vi "TestResult.vi"(0 "Name":string, 1 "Value":string, 2 "StandardValue":string, 3 "Unit":string, 4 "LowerLimit":string, 5 "UpperLimit":string, 6 "Status":T2(ring), 7 "Result":string, 8 "ProductName":string, 10 "toolID":string) -> (14 "TestIteams":T1[](array[typedef]), 15 "TestIteams2":T1[](array[typedef]))   [LabVIEW 2024]
uses:
  Ctr/TestItems.ctl
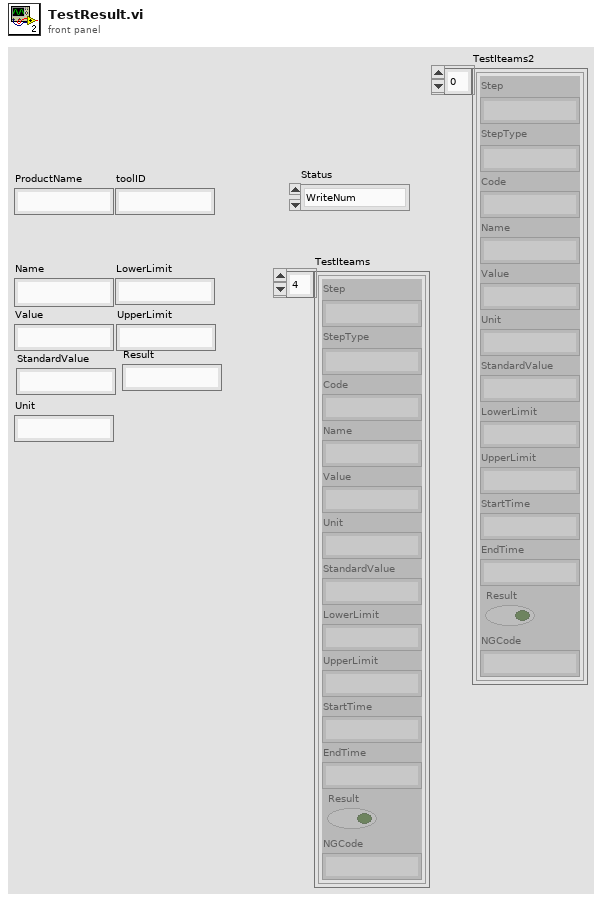
[diagram p1: front panel]
types:
  T1 = typedef "TestItems.ctl" = cluster{"Step":string, "StepType":string, "Code":string, "Name":string, "Value":string, "Unit":string, "StandardValue":string, "LowerLimit":string, "UpperLimit":string, "StartTime":string, "EndTime":string, "Result":bool, "NGCode":string}
  T2 = enum16{"WriteNum", "WriteString", "Read", "initial", "WriteNum2", "WriteString2", "Read2", "initial2"}
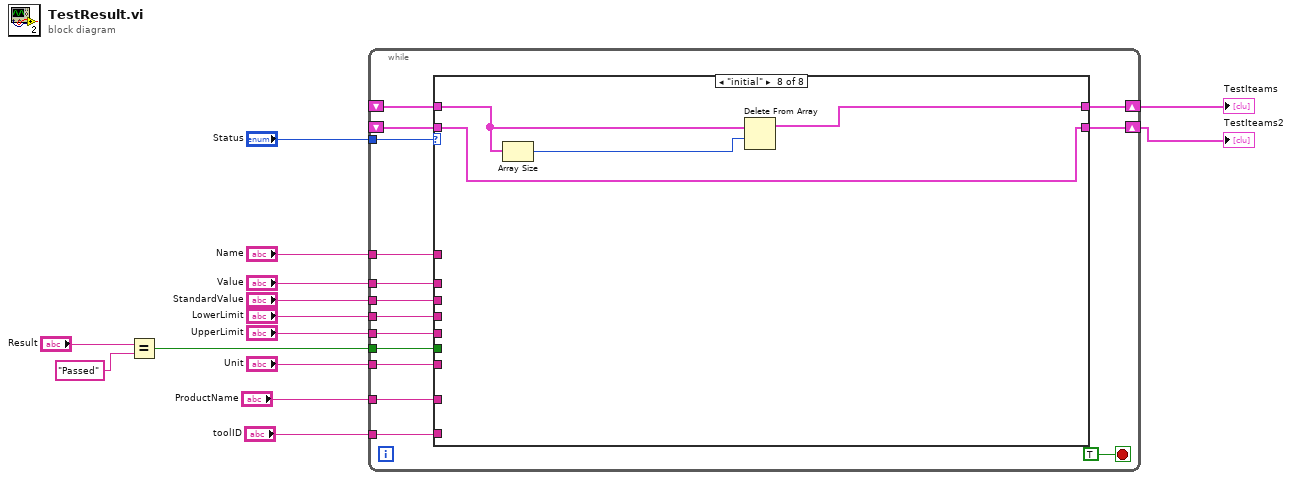
[diagram p0: block diagram]
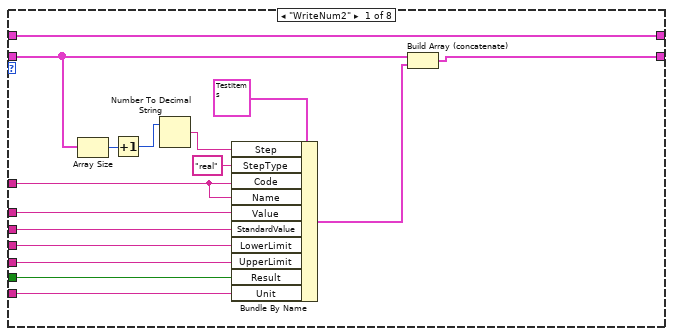
[diagram p2: hidden frame]
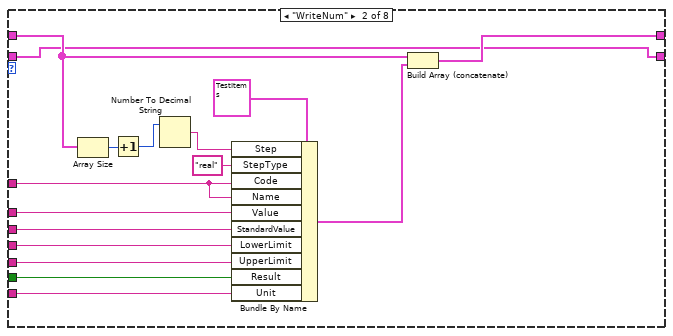
[diagram p3: hidden frame]
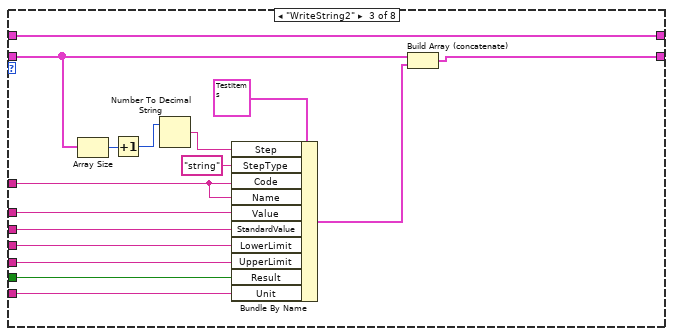
[diagram p4: hidden frame]
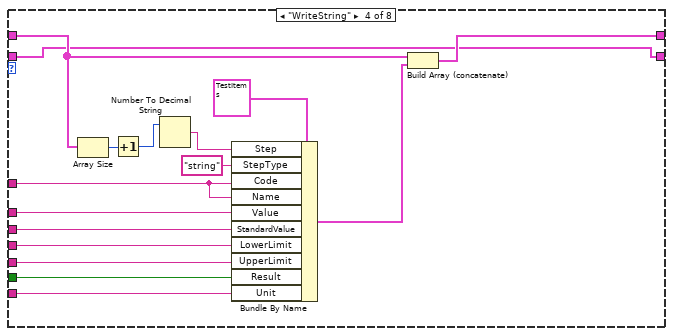
[diagram p5: hidden frame]
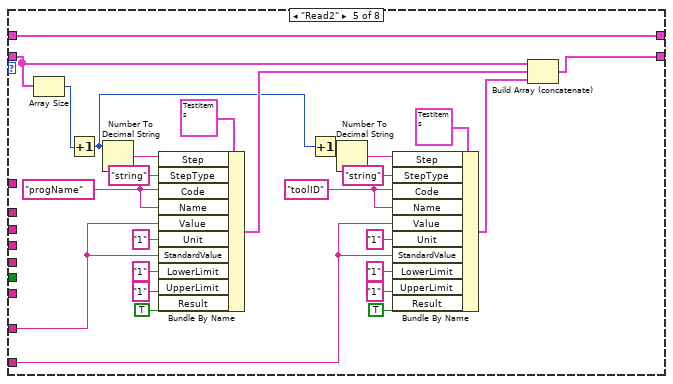
[diagram p6: hidden frame]
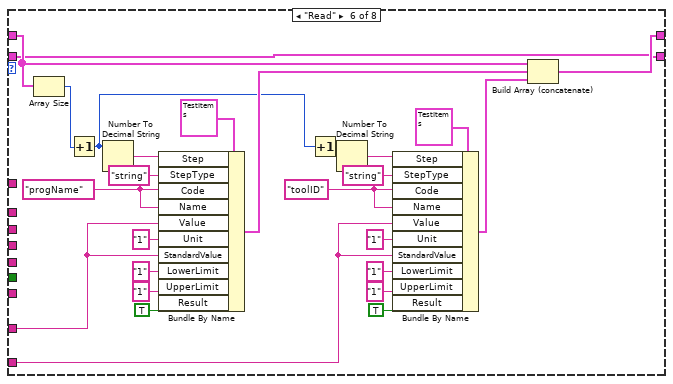
[diagram p7: hidden frame]
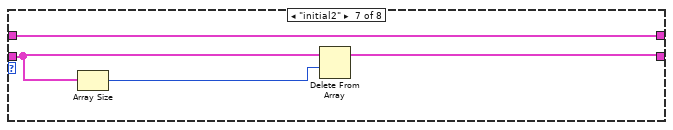
[diagram p8: hidden frame]
diagram:
  n1 = Equal?(x="Result", y="Passed") -> (x = y?=w4:bool)
  n2 = while {
    tunnel: "Status" -> [w28]
    shift-right: [w18] -> w7
    shift-left: _ -> [w17]
    tunnel: "Name" -> [w27]
    tunnel: "Value" -> [w26]
    tunnel: "StandardValue" -> [w25]
    tunnel: "LowerLimit" -> [w24]
    tunnel: "UpperLimit" -> [w23]
    tunnel: w4 -> [w22]
    tunnel: "Unit" -> [w21]
    tunnel: "ProductName" -> [w20]
    tunnel: "toolID" -> [w19]
    shift-right: [w16] -> w1
    shift-left: _ -> [w15]
    stop <- TRUE stop-if-true
    n3 = case shown="\"initial\"" w28 {
      tunnel: [w31 w47 w62 w79 w95 w121 w148 w151] -> w18
      tunnel: w17 -> [w31 w48 w62 w80 w95 w122 w148 w152]
      tunnel: w27 -> [w39 w55 w71 w87 _ _ _ _]
      tunnel: w26 -> [w38 w54 w70 w86 _ _ _ _]
      tunnel: w25 -> [w37 w53 w69 w85 _ _ _ _]
      tunnel: w24 -> [w36 w52 w68 w84 _ _ _ _]
      tunnel: w23 -> [w35 w51 w67 w83 _ _ _ _]
      tunnel: w22 -> [w34 w50 w66 w82 _ _ _ _]
      tunnel: w21 -> [w33 w49 w65 w81 _ _ _ _]
      tunnel: w20 -> [_ _ _ _ w98 w124 _ _]
      tunnel: w19 -> [_ _ _ _ w97 w123 _ _]
      tunnel: [w32 w46 w63 w78 w94 w120 w146 w150] -> w16
      tunnel: w15 -> [w30 w46 w64 w78 w96 w120 w147 w150]
      frame "WriteNum2" {
        n4 = Array Size(array=w30) -> (size(s)=w43:i32)
        n5 = Increment(x=w43) -> (x+1=w42:i32)
        n6 = Number To Decimal String(number=w42) -> (decimal integer string=w41:string)  [unwired: 1 in]
        n7 = Bundle By Name(cluster=T1 {"Step"="", "StepType"="", "Code"="", "Name"="", "Value"="", "Unit"="", "StandardValue"="", "LowerLimit"="", "UpperLimit"="", "StartTime"="", "EndTime"="", "Result"=FALSE, "NGCode"=""} ("TestItems"), "Step"=w41, "StepType"="real", "Code"=w39, "Name"=w39, "Value"=w38, "StandardValue"=w37, "LowerLimit"=w36, "UpperLimit"=w35, "Result"=w34, "Unit"=w33) -> (w44:T1)
        n8 = Build Array (concatenate)(w30, w44) -> (w32:T1[])
      }
      frame "WriteNum" {
        n9 = Array Size(array=w48) -> (size(s)=w59:i32)
        n10 = Increment(x=w59) -> (x+1=w58:i32)
        n11 = Number To Decimal String(number=w58) -> (decimal integer string=w57:string)  [unwired: 1 in]
        n12 = Bundle By Name(cluster=T1 {"Step"="", "StepType"="", "Code"="", "Name"="", "Value"="", "Unit"="", "StandardValue"="", "LowerLimit"="", "UpperLimit"="", "StartTime"="", "EndTime"="", "Result"=FALSE, "NGCode"=""} ("TestItems"), "Step"=w57, "StepType"="real", "Code"=w55, "Name"=w55, "Value"=w54, "StandardValue"=w53, "LowerLimit"=w52, "UpperLimit"=w51, "Result"=w50, "Unit"=w49) -> (w60:T1)
        n13 = Build Array (concatenate)(w48, w60) -> (w47:T1[])
      }
      frame "WriteString2" {
        n14 = Array Size(array=w64) -> (size(s)=w75:i32)
        n15 = Increment(x=w75) -> (x+1=w74:i32)
        n16 = Number To Decimal String(number=w74) -> (decimal integer string=w73:string)  [unwired: 1 in]
        n17 = Bundle By Name(cluster=T1 {"Step"="", "StepType"="", "Code"="", "Name"="", "Value"="", "Unit"="", "StandardValue"="", "LowerLimit"="", "UpperLimit"="", "StartTime"="", "EndTime"="", "Result"=FALSE, "NGCode"=""} ("TestItems"), "Step"=w73, "StepType"="string", "Code"=w71, "Name"=w71, "Value"=w70, "StandardValue"=w69, "LowerLimit"=w68, "UpperLimit"=w67, "Result"=w66, "Unit"=w65) -> (w76:T1)
        n18 = Build Array (concatenate)(w64, w76) -> (w63:T1[])
      }
      frame "WriteString" {
        n19 = Array Size(array=w80) -> (size(s)=w91:i32)
        n20 = Increment(x=w91) -> (x+1=w90:i32)
        n21 = Number To Decimal String(number=w90) -> (decimal integer string=w89:string)  [unwired: 1 in]
        n22 = Bundle By Name(cluster=T1 {"Step"="", "StepType"="", "Code"="", "Name"="", "Value"="", "Unit"="", "StandardValue"="", "LowerLimit"="", "UpperLimit"="", "StartTime"="", "EndTime"="", "Result"=FALSE, "NGCode"=""} ("TestItems"), "Step"=w89, "StepType"="string", "Code"=w87, "Name"=w87, "Value"=w86, "StandardValue"=w85, "LowerLimit"=w84, "UpperLimit"=w83, "Result"=w82, "Unit"=w81) -> (w92:T1)
        n23 = Build Array (concatenate)(w80, w92) -> (w79:T1[])
      }
      frame "Read2" {
        w105 = "toolID" ("Code")
        w115 = "progName" ("Code")
        n24 = Array Size(array=w96) -> (size(s)=w118:i32)
        n25 = Increment(x=w118) -> (x+1=w100:i32)
        n26 = Number To Decimal String(number=w100) -> (decimal integer string=w117:string)  [unwired: 1 in]
        n27 = Bundle By Name(cluster=T1 {"Step"="", "StepType"="", "Code"="", "Name"="", "Value"="", "Unit"="", "StandardValue"="", "LowerLimit"="", "UpperLimit"="", "StartTime"="", "EndTime"="", "Result"=FALSE, "NGCode"=""} ("TestItems"), "Step"=w117, "StepType"="string", "Code"=w115, "Name"=w115, "Value"=w98, "Unit"="1", "StandardValue"=w98, "LowerLimit"="1", "UpperLimit"="1", "Result"=TRUE) -> (w110:T1)
        n28 = Increment(x=w100) -> (x+1=w102:i32)
        n29 = Number To Decimal String(number=w102) -> (decimal integer string=w103:string)  [unwired: 1 in]
        n30 = Bundle By Name(cluster=T1 {"Step"="", "StepType"="", "Code"="", "Name"="", "Value"="", "Unit"="", "StandardValue"="", "LowerLimit"="", "UpperLimit"="", "StartTime"="", "EndTime"="", "Result"=FALSE, "NGCode"=""} ("TestItems"), "Step"=w103, "StepType"="string", "Code"=w105, "Name"=w105, "Value"=w97, "Unit"="1", "StandardValue"=w97, "LowerLimit"="1", "UpperLimit"="1", "Result"=TRUE) -> (w99:T1)
        n31 = Build Array (concatenate)(w96, w110, w99) -> (w94:T1[])
      }
      frame "Read" {
        w131 = "toolID" ("Code")
        w141 = "progName" ("Code")
        n32 = Array Size(array=w122) -> (size(s)=w144:i32)
        n33 = Increment(x=w144) -> (x+1=w126:i32)
        n34 = Number To Decimal String(number=w126) -> (decimal integer string=w143:string)  [unwired: 1 in]
        n35 = Bundle By Name(cluster=T1 {"Step"="", "StepType"="", "Code"="", "Name"="", "Value"="", "Unit"="", "StandardValue"="", "LowerLimit"="", "UpperLimit"="", "StartTime"="", "EndTime"="", "Result"=FALSE, "NGCode"=""} ("TestItems"), "Step"=w143, "StepType"="string", "Code"=w141, "Name"=w141, "Value"=w124, "Unit"="1", "StandardValue"=w124, "LowerLimit"="1", "UpperLimit"="1", "Result"=TRUE) -> (w136:T1)
        n36 = Increment(x=w126) -> (x+1=w128:i32)
        n37 = Number To Decimal String(number=w128) -> (decimal integer string=w129:string)  [unwired: 1 in]
        n38 = Bundle By Name(cluster=T1 {"Step"="", "StepType"="", "Code"="", "Name"="", "Value"="", "Unit"="", "StandardValue"="", "LowerLimit"="", "UpperLimit"="", "StartTime"="", "EndTime"="", "Result"=FALSE, "NGCode"=""} ("TestItems"), "Step"=w129, "StepType"="string", "Code"=w131, "Name"=w131, "Value"=w123, "Unit"="1", "StandardValue"=w123, "LowerLimit"="1", "UpperLimit"="1", "Result"=TRUE) -> (w125:T1)
        n39 = Build Array (concatenate)(w122, w136, w125) -> (w121:T1[])
      }
      frame "initial2" {
        n40 = Array Size(array=w147) -> (size(s)=w149:i32)
        n41 = Delete From Array(array=w147, length=w149) -> (array with subset deleted=w146:T1[])  [unwired: 1 in, 1 out]
      }
      frame "initial" {
        n42 = Array Size(array=w152) -> (size(s)=w153:i32)
        n43 = Delete From Array(array=w152, length=w153) -> (array with subset deleted=w151:T1[])  [unwired: 1 in, 1 out]
      }
    }
  }
  "TestIteams" <- w7
  "TestIteams2" <- w1
